vi "setSnakeStartPoint.vi"(4 "StartPointY":i32, 6 "StartPointX":i32, 8 "error in (no error)":errorcluster, 11 "Snake in":refnum<class "Snake.lvclass">) -> (0 "error out":errorcluster, 3 "Snake out":refnum<class "Snake.lvclass">)   [LabVIEW 2014, in "Snake.lvclass"]
uses:
  Snake.lvclass
  Snake.lvclass/Snake.ctl
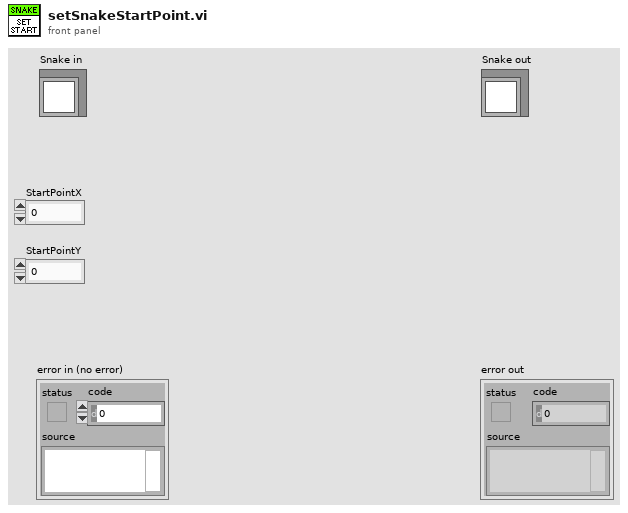
[diagram p1: front panel]
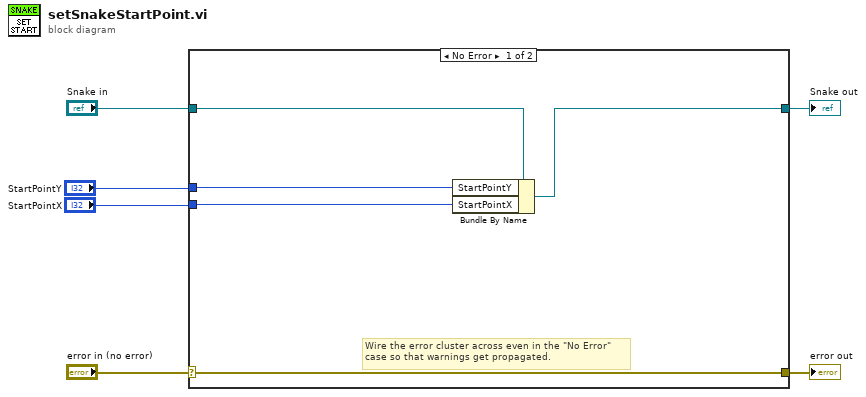
[diagram p0: block diagram]
diagram:
  n1 = case shown="No Error" "error in (no error)" {
    selector: "error in (no error)" -> [w11 w13]
    tunnel: [w11 w13] -> w5
    tunnel: [w9 w12] -> w3
    tunnel: "Snake in" -> [w10 w12]
    tunnel: "StartPointY" -> [w8 _]
    tunnel: "StartPointX" -> [w7 _]
    frame No Error {
      # "Wire the error cluster across even in the \"No Error\"\ncase so that warnings get propagated."
      n2 = Bundle By Name(cluster=w10, "StartPointY"=w8, "StartPointX"=w7) -> (w9:refnum<class "Snake.lvclass">)
    }
    frame Error {
    }
  }
  "error out" <- w5
  "Snake out" <- w3
